vi "launch_main.vi"(8 "error in (no error)":errorcluster, 10 "queue_size":i32=10, 11 "run_f_stop_t":bool) -> (0 "error out":errorcluster)   [LabVIEW 2015, in "lv-recipe-machine.lvlib"]
doc: "launch_main.vi is a kind of functional global that can be used to start or stop the main of the recipe_machine module. It has an internal feedback node to store the vi reference once started and uses a queue to retrieve the references upon successful start."
uses:
  lv-recipe-machine.lvlib
  _controls/fg_command.ctl
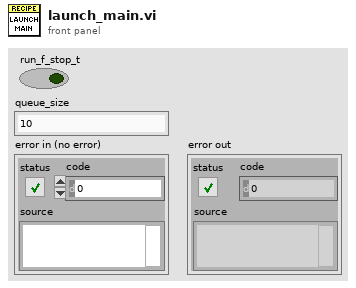
[diagram p1: front panel]
types:
  T1 = typedef "lv-recipe-machine.lvlib/fg_command.ctl" = enum16{"<fg_command>", "initialize", "read", "write", "shutdown", "<null>"}
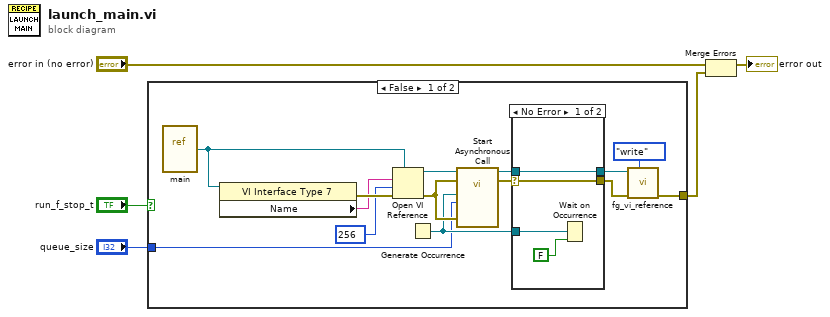
[diagram p0: block diagram]
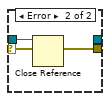
[diagram p2: hidden frame]
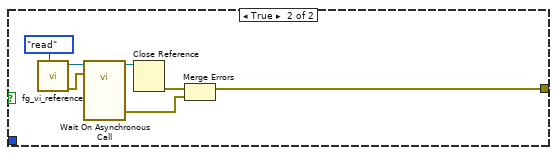
[diagram p3: hidden frame]
diagram:
  n1 = case shown="False" "run_f_stop_t" {
    tunnel: [w8 w30] -> w3
    tunnel: "queue_size" -> [w10 _]
    frame False {
      n2 = vi-ref "main.vi"() -> (w14:refnum<vi>)
      n3 = property class="VI Interface Type 7"(reference=w14) -> (error out=w19:errorcluster, "Name"=w18:string)  [unwired: 1 in, 1 out]
      n4 = Open VI Reference(type specifier VI Refnum (for type only)=w14, vi path=w18, options=256, error in (no error)=w19) -> (vi reference=w13:refnum<vi>, error out=w12:errorcluster)  [unwired: 2 in]
      n5 = Generate Occurrence() -> (w11:refnum<k4>)
      n6 = call-by-ref "Start Asynchronous Call"(reference=w13, error in=w12, 8:"error in (no error)"=w12, "max_queue_size"=w10, "occurrence"=w11) -> (reference out=w15:refnum<vi>, error out=w16:errorcluster)  [unwired: 8 in, 1 out]
      n7 = case shown="No Error" w16 {
        selector: w16 -> [w20 w25]
        tunnel: [w20 w25] -> w9
        tunnel: w15 -> [w23 w24]
        tunnel: [w23 _] -> w7
        tunnel: w11 -> [w22 _]
        frame No Error {
          n8 = Wait on Occurrence(1:FALSE ("ignore previous (T)"), 2:w22) -> ()  [unwired: 1 in, 1 out]
        }
        frame Error {
          n9 = Close Reference(reference=w24) -> ()  [unwired: 1 in, 1 out]
        }
      }
      n10 = call "fg_vi_reference.vi"("command"=fg_command."write", "error in (no error)"=w9, "vi_reference in"=w7) -> ("error out"=w8:errorcluster)  [unwired: 7 in, 1 out]
    }
    frame True {
      n11 = call "fg_vi_reference.vi"("command"=fg_command."read") -> ("error out"=w26:errorcluster, "vi_reference out"=w27:refnum<vi>)  [unwired: 9 in]
      n12 = call-by-ref "Wait On Asynchronous Call"(reference=w27, error in=w26) -> (reference out=w32:refnum<vi>, "error out"=w29:errorcluster)  [unwired: 11 in, 1 out]
      n13 = Close Reference(reference=w32) -> (error out=w31:errorcluster)  [unwired: 1 in]
      n14 = Merge Errors(w31, w29) -> (w30:errorcluster)
    }
  }
  n15 = Merge Errors("error in (no error)", w3) -> (→"error out":errorcluster)
